vi "mod T params primary.vi"(2 "Set T params":bool, 7 "exp exec in":T1={"data file"={"autosave"=FALSE, "File refnum"=refnum, "data file path"=path ""}, "T log file"={"File refnum"=refnum, "T log file path"=path "", "exists"=FALSE}, "exp seq"={"wave params"={"Num of avg"=584, "Num points"=1000, "Meas rate (Hz)"=100000.0}, "Setpoints"=[], "#"=-1, "index"=-1, "elapsed time (s)"=0.0, "set time (s)"=0.0, "min settle (s)"=30.0, " Exec Status"=enum."Settling"}, "error"={"status"=FALSE, "code"=0, "source"=""}}) -> (8 "exp exec out":T1={"data file"={"autosave"=FALSE, "File refnum"=refnum, "data file path"=path ""}, "T log file"={"File refnum"=refnum, "T log file path"=path "", "exists"=FALSE}, "exp seq"={"wave params"={"Num of avg"=584, "Num points"=1000, "Meas rate (Hz)"=100000.0}, "Setpoints"=[], "#"=-1, "index"=-1, "elapsed time (s)"=0.0, "set time (s)"=0.0, "min settle (s)"=30.0, " Exec Status"=enum."Settling"}, "error"={"status"=FALSE, "code"=0, "source"=""}})   [LabVIEW 2019]
doc: "This is a Bug C(T) subVI.\n\nIt is a shell for a popup that allows the user to modify the temp control parameters from the initialization loop.\n\nPaul K Dixon\nP3600\nCSUSB Physics"
uses:
  typedefs/PID exec cluster.ctl
  typedefs/data file info.ctl
  typedefs/bug temp file info.ctl
  typedefs/exp seq cluster.ctl
  typedefs/wvfm acq params.ctl
  typedefs/bug meas status.ctl
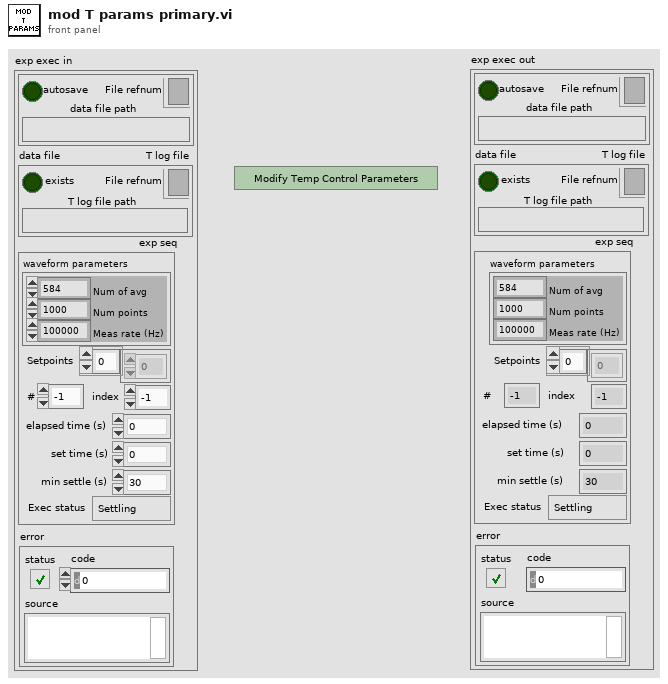
[diagram p1: front panel]
types:
  T1 = typedef "PID exec cluster.ctl" = cluster{"data file":T2, "T log file":T3, "exp seq":T4, "error":errorcluster}
  T2 = typedef "data file info.ctl" = cluster{"autosave":bool, "File refnum":refnum<file>, "data file path":path}
  T3 = typedef "bug temp file info.ctl" = cluster{"File refnum":refnum<file>, "T log file path":path, "exists":bool}
  T4 = typedef "exp seq cluster.ctl" = cluster{"wave params":T5, "Setpoints":dbl[], "#":i32, "index":i32, "elapsed time (s)":dbl, "set time (s)":dbl, "min settle (s)":dbl, " Exec Status":T6}
  T5 = typedef "wvfm acq params.ctl" = cluster{"Num of avg":i32, "Num points":i32, "Meas rate (Hz)":dbl}
  T6 = typedef "bug meas status.ctl" = enum32{"Settling", "Measuring", "Holding", "Exit"}
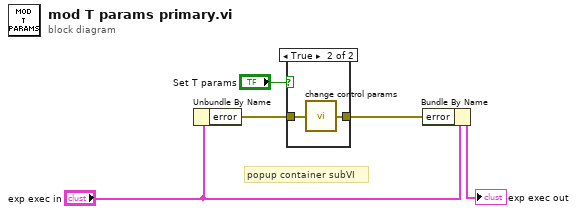
[diagram p0: block diagram]
diagram:
  # "popup container subVI"
  n1 = Unbundle By Name("exp exec in") -> ("error"=w4:errorcluster)
  n2 = case shown="True" "Set T params" {
    tunnel: w4 -> [w6 w8]
    tunnel: [w6 w7] -> w3
    frame False {
    }
    frame True {
      n3 = call "change control params.vi"("exp exec in"=w8) -> ("exp exec in"=w7:errorcluster)  [unwired: 14 in]
    }
  }
  n4 = Bundle By Name(cluster="exp exec in", "error"=w3) -> (→"exp exec out":T1)
